vi "SetRobotProfile.vi"   [LabVIEW 2020]
doc: "Reads the robot profile from the configuration file on the roboRIO and sets any robot specific parameters."
uses:
  GlobalMiscellaneous.vi
  GlobalDrivebase.vi
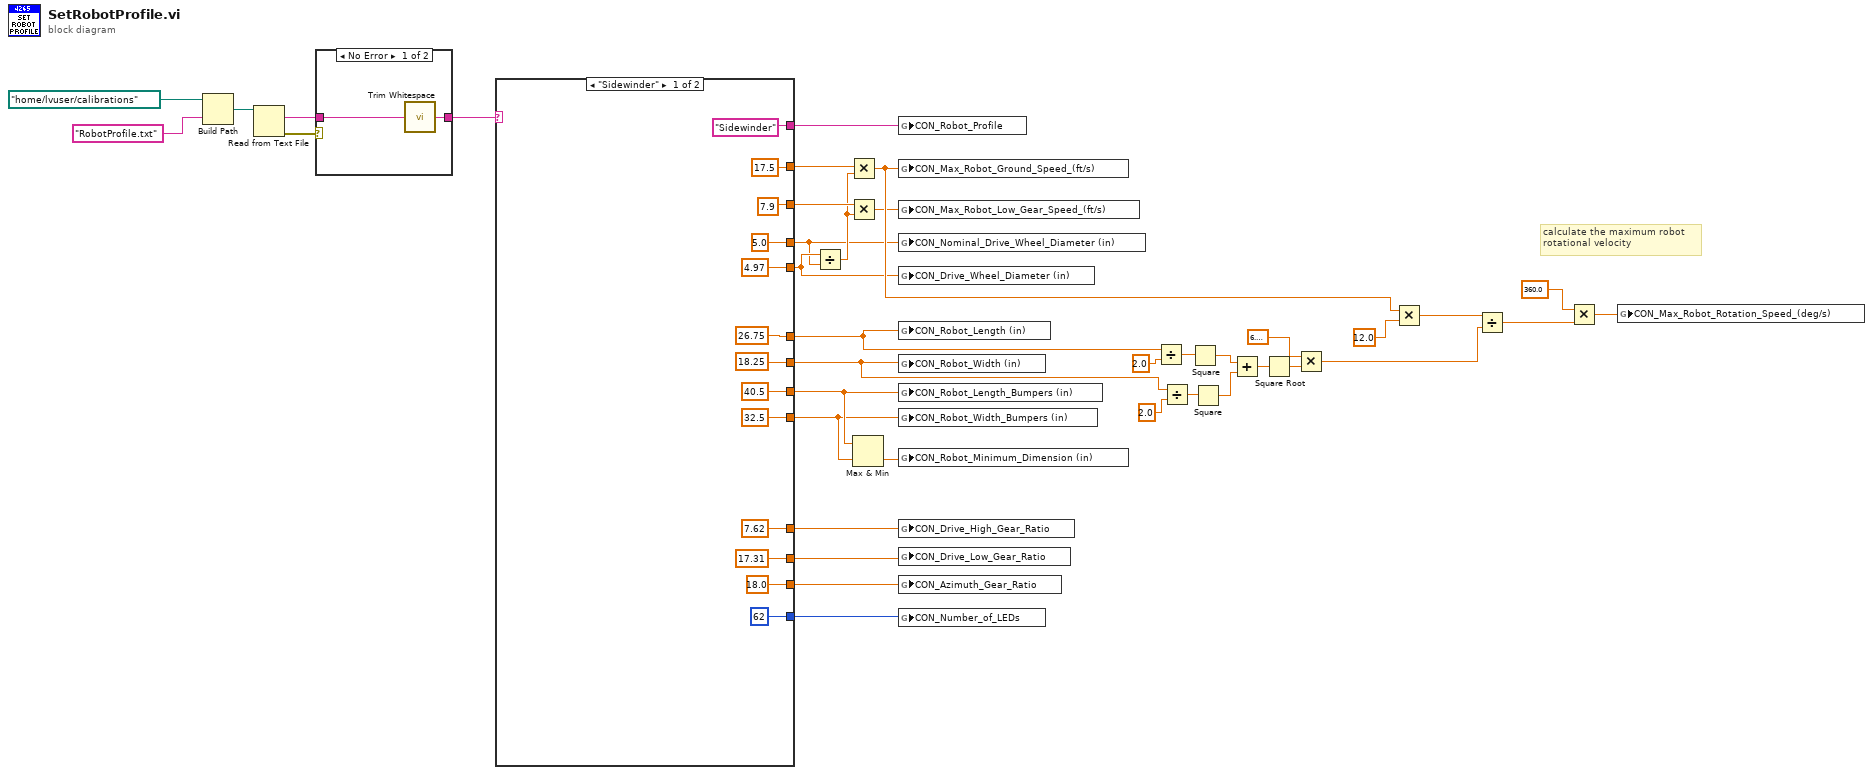
[diagram p0: block diagram]
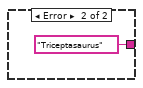
[diagram p2: hidden frame]
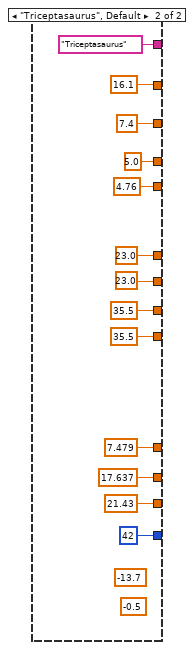
[diagram p3: hidden frame]
diagram:
  # "calculate the maximum robot\nrotational velocity"
  n1 = Build Path(base path=path "/home/lvuser/calibrations" ("path"), name or relative path="RobotProfile.txt") -> (appended path=w37:path)
  n2 = Read from Text File(file (use dialog)=w37) -> (text=w35:string, error out=w36:errorcluster)  [unwired: 3 in, 2 out]
  n3 = case shown="No Error" w36 {
    tunnel: w35 -> [w39 _]
    tunnel: [w40 "Triceptasaurus"] -> w33
    frame No Error {
      n4 = call <vilib>:"Trim Whitespace.vi"("string"=w39) -> ("trimmed string"=w40:string)  [unwired: 1 in]
    }
    frame Error {
    }
  }
  n5 = case shown="\"Sidewinder\"" w33 {
    tunnel: ["Sidewinder" "Triceptasaurus"] -> w8
    tunnel: [18.25 ("Robot_Length (in)") 23.0 ("Robot_Length (in)")] -> w17
    tunnel: [26.75 ("Robot_Length (in)") 23.0 ("Robot_Length (in)")] -> w18
    tunnel: [17.5 ("Max_Robot_Ground_Speed_(ft/s)") 16.1 ("Max_Robot_Ground_Speed_(ft/s)")] -> w7
    tunnel: [40.5 ("Robot_Length (in)") 35.5 ("Robot_Length (in)")] -> w16
    tunnel: [32.5 ("Robot_Length (in)") 35.5 ("Robot_Length (in)")] -> w15
    tunnel: [5.0 ("Robot_Length (in)") 5.0 ("Robot_Length (in)")] -> w1
    tunnel: [7.62 ("Robot_Length (in)") 7.479 ("Robot_Length (in)")] -> w13
    tunnel: [17.31 ("Robot_Length (in)") 17.637 ("Robot_Length (in)")] -> w12
    tunnel: [18.0 ("Robot_Length (in)") 21.43 ("Robot_Length (in)")] -> w11
    tunnel: [u16 62 u16 42] -> w9
    tunnel: [7.9 ("Max_Robot_Ground_Speed_(ft/s)") 7.4 ("Max_Robot_Ground_Speed_(ft/s)")] -> w5
    tunnel: [4.97 ("Robot_Length (in)") 4.76 ("Robot_Length (in)")] -> w2
    frame "Sidewinder" {
    }
    frame "Triceptasaurus", Default {
      (unwired) -0.5
      (unwired) -13.7
    }
  }
  n6 = Divide(x=w2, y=w1) -> (x/y=w3:dbl)
  n7 = Multiply(x=w7, y=w3) -> (x*y=w6:dbl)
  n8 = Multiply(x=w5, y=w3) -> (x*y=w4:dbl)
  n9 = Max & Min(x=w16, y=w15) -> (min(x,y)=w14:dbl)  [unwired: 1 out]
  n10 = global write "GlobalMiscellaneous.vi" "CON_Robot_Profile"(w8) -> ()
  n11 = global write "GlobalDrivebase.vi" "CON_Max_Robot_Ground_Speed_(ft/s)"(w6) -> ()
  n12 = global write "GlobalDrivebase.vi" "CON_Max_Robot_Low_Gear_Speed_(ft/s)"(w4) -> ()
  n13 = global write "GlobalDrivebase.vi" "CON_Nominal_Drive_Wheel_Diameter (in)"(w1) -> ()
  n14 = global write "GlobalDrivebase.vi" "CON_Drive_Wheel_Diameter (in)"(w2) -> ()
  n15 = global write "GlobalDrivebase.vi" "CON_Robot_Length (in)"(w18) -> ()
  n16 = global write "GlobalDrivebase.vi" "CON_Robot_Width (in)"(w17) -> ()
  n17 = global write "GlobalDrivebase.vi" "CON_Robot_Length_Bumpers (in)"(w16) -> ()
  n18 = global write "GlobalDrivebase.vi" "CON_Robot_Width_Bumpers (in)"(w15) -> ()
  n19 = global write "GlobalDrivebase.vi" "CON_Robot_Minimum_Dimension (in)"(w14) -> ()
  n20 = global write "GlobalDrivebase.vi" "CON_Drive_High_Gear_Ratio"(w13) -> ()
  n21 = global write "GlobalDrivebase.vi" "CON_Drive_Low_Gear_Ratio"(w12) -> ()
  n22 = global write "GlobalDrivebase.vi" "CON_Azimuth_Gear_Ratio"(w11) -> ()
  n23 = global write "GlobalMiscellaneous.vi" "CON_Number_of_LEDs"(w9) -> ()
  n24 = Divide(x=w18, y=2.0) -> (x/y=w24:dbl)
  n25 = Divide(x=w17, y=2.0) -> (x/y=w23:dbl)
  n26 = Square(x=w24) -> (x^2=w22:dbl)
  n27 = Square(x=w23) -> (x^2=w21:dbl)
  n28 = Add(x=w22, y=w21) -> (x+y=w20:dbl)
  n29 = Square Root(x=w20) -> (sqrt(x)=w19:dbl)
  n30 = Multiply(x=6.283185307179586, y=w19) -> (x*y=w29:dbl)
  n31 = Multiply(x=w6, y=12.0) -> (x*y=w31:dbl)
  n32 = Divide(x=w31, y=w29) -> (x/y=w28:dbl)
  n33 = Multiply(x=360.0, y=w28) -> (x*y=w10:dbl)
  n34 = global write "GlobalDrivebase.vi" "CON_Max_Robot_Rotation_Speed_(deg/s)"(w10) -> ()
